vi "influxdb.vi"() -> ()   [LabVIEW 2023]
uses:
  <vilib>/httpClient/POSTBuffer.vi
  <vilib>/httpClient/LabVIEWHTTPClient.lvlib
panel:
  out "error out":errorcluster
  in  "error in (no error)":errorcluster
  out "body 2":string
  out "body 3":string
  out "body":string
  # "Quickie Influxdb interface using http posts & buffers"
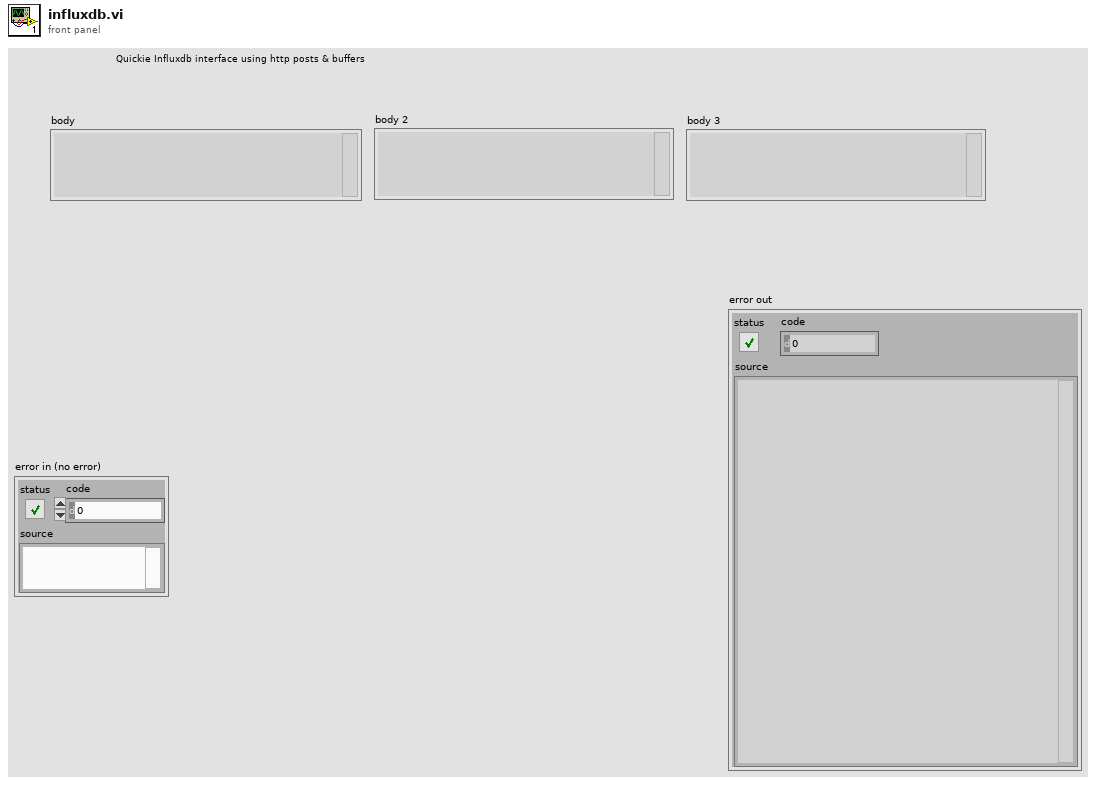
[diagram p1: front panel]
types:
  T1 = typedef "LabVIEWHTTPClient.lvlib/ClientHandle.ctl" = refnum<k1>
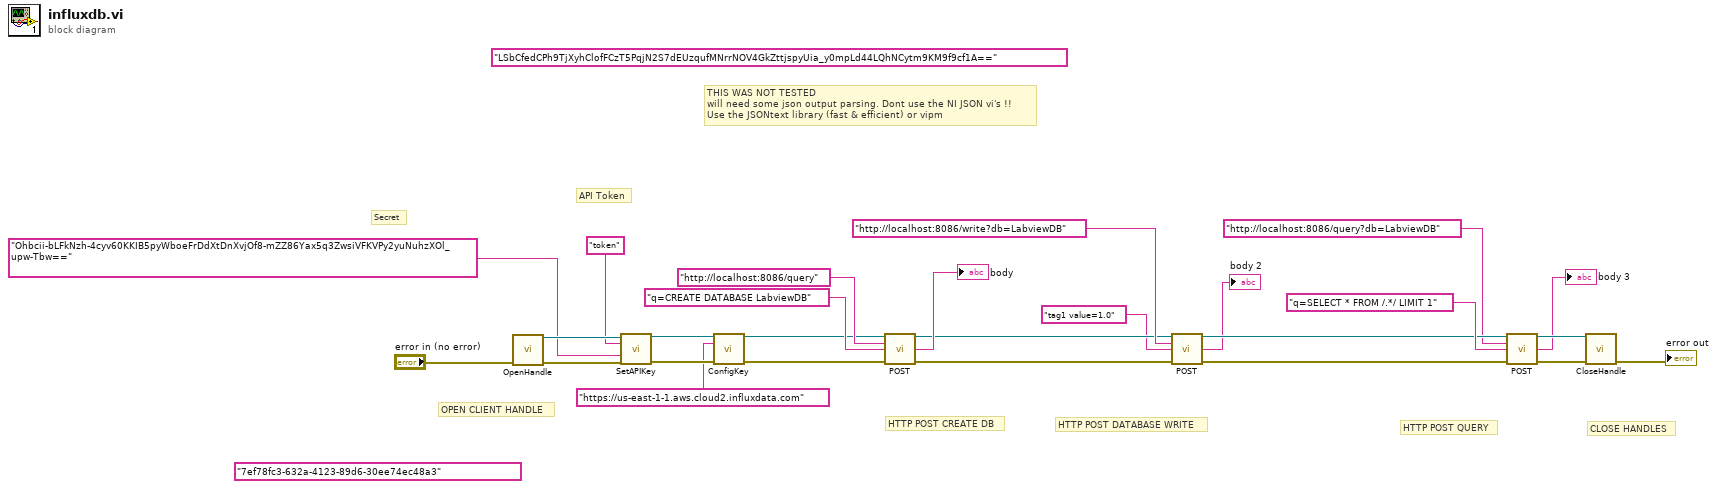
[diagram p0: block diagram]
diagram:
  (unwired) "7ef78fc3-632a-4123-89d6-30ee74ec48a3"
  (unwired) "LSbCfedCPh9TjXyhClofFCzT5PqjN2S7dEUzqufMNrrNOV4GkZttjspyUia_y0mpLd44LQhNCytm9KM9f9cf1A=="
  # "API Token"
  # "Secret"
  # "THIS WAS NOT TESTED\nwill need some json output parsing. Dont use the NI JSON vi's !!\nUse the JSONtext library (fast & efficient) or vipm"
  # "CLOSE HANDLES"
  # "HTTP POST QUERY"
  # "HTTP POST DATABASE WRITE"
  # "HTTP POST CREATE DB"
  # "OPEN CLIENT HANDLE"
  n1 = call <vilib>:"OpenHandle.vi"("error in (no error)"="error in (no error)") -> ("client handle out"=w9:T1, "error out"=w8:errorcluster)  [unwired: 13 in]
  n2 = call <vilib>:"SetAPIKey.vi"("client handle"=w9, "access id"="token", "secret id"="Ohbcii-bLFkNzh-4cyv60KKIB5pyWboeFrDdXtDnXvjOf8-mZZ86Yax5q3ZwsiVFKVPy2yuNuhzXOl_upw-Tbw==", "error in (no error)"=w8) -> ("client handle out"=w5:T1, "error out"=w3:errorcluster)  [unwired: 10 in]
  n3 = call <vilib>:"ConfigKey.vi"("client handle"=w5, "host"="https://us-east-1-1.aws.cloud2.influxdata.com", "error in (no error)"=w3) -> ("client handle out"=w4:T1, "error out"=w2:errorcluster)  [unwired: 11 in]
  n4 = call-poly <vilib>:"POST.vi"("client handle"=w4, "url"="http://localhost:8086/query", "buffer"="q=CREATE DATABASE LabviewDB" ("Query String"), "error in (no error)"=w2) -> ("client handle out"=w18:T1, "body"=→"body":string, "error out"=w16:errorcluster)  [unwired: 8 in, 1 out]
  n5 = call-poly <vilib>:"POST.vi"("client handle"=w18, "url"="http://localhost:8086/write?db=LabviewDB", "buffer"="tag1 value=1.0", "error in (no error)"=w16) -> ("client handle out"=w17:T1, "body"=→"body 2":string, "error out"=w15:errorcluster)  [unwired: 8 in, 1 out]
  n6 = call-poly <vilib>:"POST.vi"("client handle"=w17, "url"="http://localhost:8086/query?db=LabviewDB", "buffer"="q=SELECT * FROM /.*/ LIMIT 1" ("Query String"), "error in (no error)"=w15) -> ("client handle out"=w23:T1, "body"=→"body 3":string, "error out"=w22:errorcluster)  [unwired: 8 in, 1 out]
  n7 = call <vilib>:"CloseHandle.vi"("client handle"=w23, "error in (no error)"=w22) -> ("error out"=→"error out":errorcluster)  [unwired: 13 in]
